vi "Untitled.vi"() -> ()   [LabVIEW 2011]
uses:
  <vilib>/Platform/TimedLoop/XDataNode/timing_clust.ctl
  <vilib>/Platform/TimedLoop/XDataNode/nitl_modes.ctl
  <vilib>/Platform/TimedLoop/XDataNode/wakeup.ctl
  <vilib>/Platform/TimedLoop/XDataNode/XDataNode.xnode
  <vilib>/Platform/TimedLoop/XDataNode/XDNodeRunTimeDep.lvlib
panel:
  in  "stop":bool
  out "Value":dbl
  out "Outcome":enum16{"RampUp", "Hold", "RampDown"}(ring)
  in  "HoldTime":u64=1000 caption="Hold Time (ms)"
  in  "RampTime":u64=1000 caption="Ramp Time (ms)"
  out "BaseCount":u64
  out "LoopCount":u64
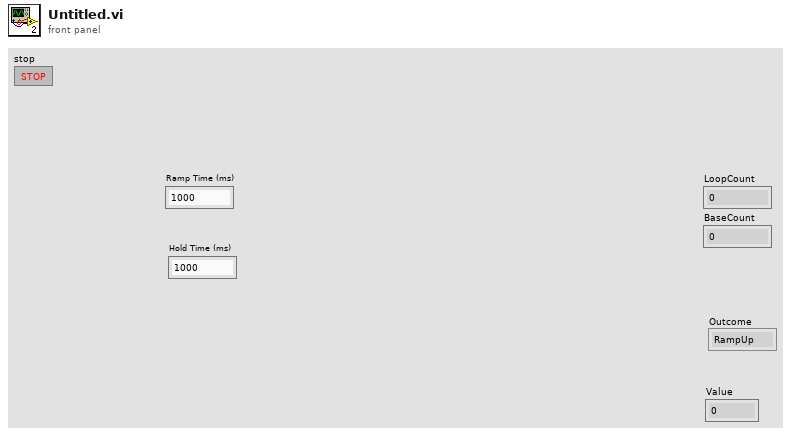
[diagram p1: front panel]
types:
  T1 = typedef "XDNodeRunTimeDep.lvlib/timing_clust.ctl" = cluster{"Expected End [f-1]":u64, "Actual End [f-1]":u64, "Finished Late? [f-1]":bool, "Expected End [i-1]":u64, "Actual End [i-1]":u64, "Finished Late? [i-1]":bool, "Expected Start [i]":u64, "Actual Start [i]":u64, "Expected Start [f]":u64, "Actual Start [f]":u64, "Source Name":string, "Structure Name":string, "Period":i64, "Deadline":i64, "Offset":i64, "Start":i64, "Priority":i32, "Timeout":i32, "Mode":T2, "Wakeup Reason":T3, "Error":errorcluster, "Source Type":string, "Secondary Source Type":string, "Global End Time":u64, "Global Start Time":u64, "Frame Duration":u64, "Iteration Duration":u64, "Assigned CPU":i32, "I/O Scan Engine Mode":u32}
  T2 = typedef "XDNodeRunTimeDep.lvlib/nitl_modes.ctl" = enum32{"No Change", "Process missed periods, maintain original phase", "Discard missed periods, maintain original phase", "Process missed periods, ignore original phase", "Discard missed periods, ignore original phase"}
  T3 = typedef "XDNodeRunTimeDep.lvlib/wakeup.ctl" = enum32{"Normal", "Aborted", "Asynchronous wakeup", "Timing source error", "Timed loop error", "Timeout"}
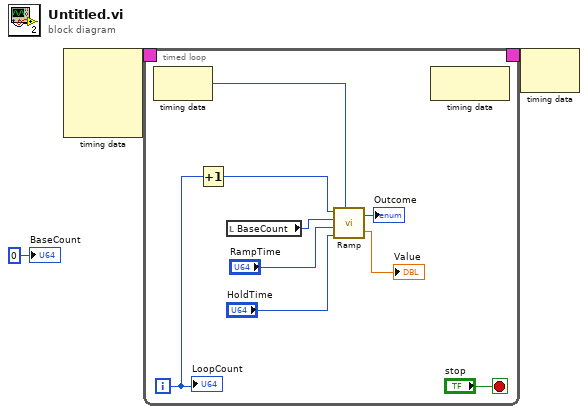
[diagram p0: block diagram]
diagram:
  n1 = node-c288() -> (w3:T1)  [unwired: 4 in]
  n2 = timed-loop {
    timing: w3 -> [_]
    timing-out: [_] -> w2
    i -> [w5]
    stop <- "stop" stop-if-true
    n3 = node-c288() -> (w9:i64)  [unwired: 1 in]
    n4 = Increment(x=w5) -> (x+1=w4:i32)
    n5 = local read "BaseCount"() -> (w12:u64)
    n6 = call "Ramp.vi"("LoopPeriod"=w9, "HoldTime"="HoldTime", "RampTime"="RampTime", "BaseCount"=w12, "LoopCount"=w4) -> ("Value"=→"Value":dbl, "Outcome"=→"Outcome":enum16{"RampUp", "Hold", "RampDown"})  [unwired: 1 in]
    n7 = node-c288() -> ()  [unwired: 1 in, 1 out]
    "LoopCount" <- w5
  }
  n8 = node-c288(w2) -> ()  [unwired: 1 out]
  "BaseCount" <- u64 0 ("BaseCount")
